vi "test_main.vi"(8 "error in (no error)":errorcluster) -> (0 "error out":errorcluster)   [LabVIEW 2023, in "horiba.test.lvlib"]
uses:
  horiba.test.lvlib
  <vilib>/addons/_JKI Toolkits/Caraya/classes/Test/Test.lvclass
panel:
  # "Connector Pane"
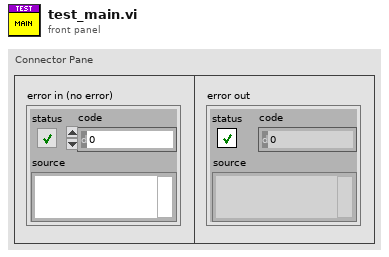
[diagram p1: front panel]
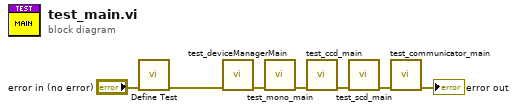
[diagram p0: block diagram]
diagram:
  n1 = call <vilib>:"Define Test.vi"("error in (no error)"="error in (no error)") -> ("error out"=w3:errorcluster)  [unwired: 9 in, 1 out]
  n2 = call "test_deviceManagerMain.vi"("error in (no error)"=w3) -> ("error out"=w6:errorcluster)  [unwired: 10 in]
  n3 = call "test_mono_main.vi"("error in"=w6) -> ("error out"=w5:errorcluster)  [unwired: 10 in]
  n4 = call "test_ccd_main.vi"("error in (no error)"=w5) -> ("error out"=w4:errorcluster)  [unwired: 10 in]
  n5 = call "test_scd_main.vi"("error in"=w4) -> ("error out"=w1:errorcluster)  [unwired: 10 in]
  n6 = call "test_communicator_main.vi"("error in (no error)"=w1) -> ("error out"=→"error out":errorcluster)  [unwired: 10 in]
